vi "Waveform Update Name and Script.vi"(0 "Waveform in":T1 {"Runtime Scaling" format="%#_6p"; "Sample Rate" format="%#_6p"; "Burst Length (s)" format="%#_6p"; "PAPR (dB)" format="%.2f"; "Signal Bandwidth (Hz)" format="%#_6p"}, 7 "New Waveform Name":string) -> (4 "Waveform out":T1 {"Runtime Scaling" format="%#_6p"; "Sample Rate" format="%#_6p"; "Burst Length (s)" format="%#_6p"; "PAPR (dB)" format="%.2f"; "Signal Bandwidth (Hz)" format="%#_6p"})   [LabVIEW 2019, in "Common.lvlib"]
doc: "Updates the <b>Name</b> value with <b>New Waveform Name</b> and replaces any reference to it in <b>Script</b>."
uses:
  Common.lvlib
  Waveform.ctl
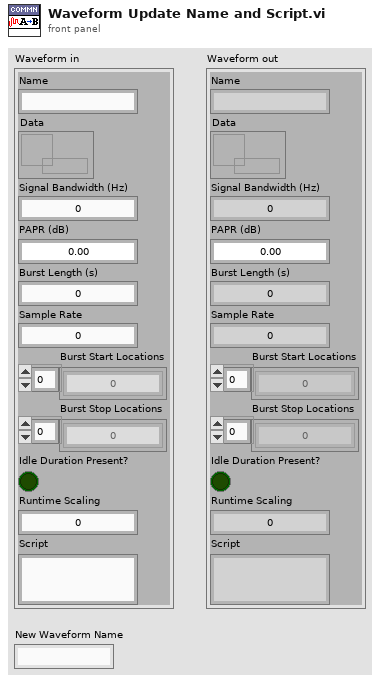
[diagram p1: front panel]
types:
  T1 = typedef "Common.lvlib/Waveform.ctl" = cluster{"Name":string, "Data":refnum<data-value>, "Signal Bandwidth (Hz)":dbl, "PAPR (dB)":dbl, "Burst Length (s)":dbl, "Sample Rate":dbl, "Burst Start Locations":i32[], "Burst Stop Locations":i32[], "Idle Duration Present?":bool, "Runtime Scaling":dbl, "Script":string}
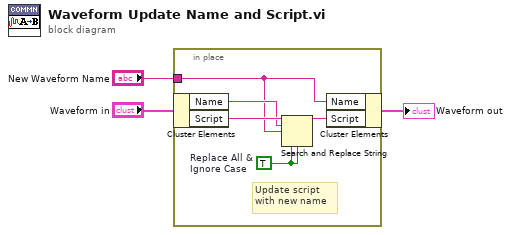
[diagram p0: block diagram]
diagram:
  n1 = in-place {
    in-place-border: "New Waveform Name" -> [w4]
    w6 = TRUE  # Replace All & Ignore Case
    # "Update script\nwith new name"
    n2 = in-place-cluster #1("Waveform in") -> ("Name"=w5:string, "Script"=w8:string)
    n3 = Search and Replace String(replace all?=w6, case sensitive?=w6, input string=w8, search string=w5, replace string=w4) -> (result string=w7:string)  [unwired: 3 in, 3 out]
    n4 = in-place-cluster #1("Name"=w4, "Script"=w7) -> (→"Waveform out":T1)
  }
